vi "Write appender queue.vi"(8 "error in (no error)":errorcluster caption="에러 입력(에러 없음)", 10 "appender queue":refnum<queue>, 11 "GUI Log Class 입력":refnum<class "GUI Log Class.lvclass">) -> (0 "error out":errorcluster caption="에러 출력", 3 "GUI Log Class 출력":refnum<class "GUI Log Class.lvclass">)   [LabVIEW 2020, in "GUI Log Class.lvclass"]
uses:
  GUI Log Class.lvclass
  GUI Log Class.lvclass/GUI Log Class.ctl
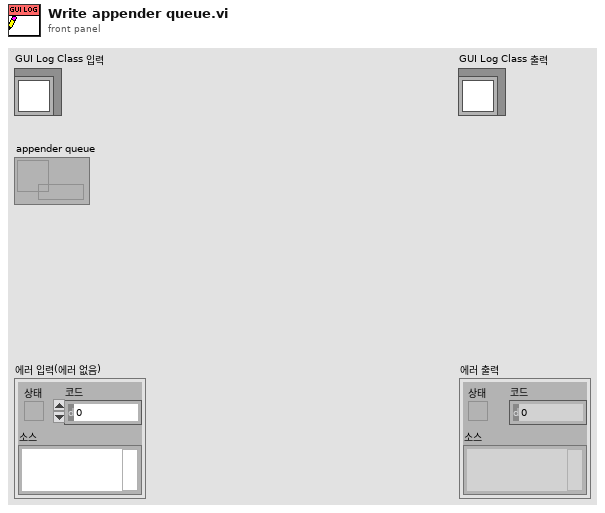
[diagram p1: front panel]
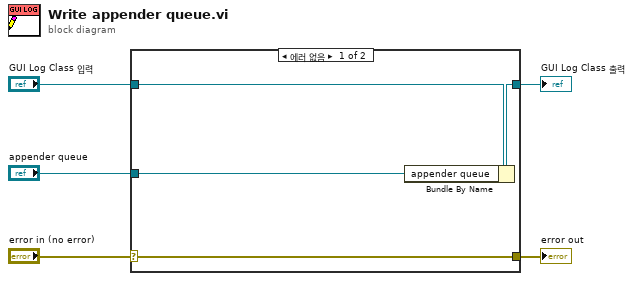
[diagram p0: block diagram]
diagram:
  n1 = case shown="에러 없음" "error in (no error)" {
    selector: "error in (no error)" -> [w9 w10]
    tunnel: [w9 w10] -> w4
    tunnel: [w7 w11] -> w2
    tunnel: "GUI Log Class 입력" -> [w8 w11]
    tunnel: "appender queue" -> [w6 _]
    frame No Error {
      n2 = Bundle By Name(cluster=w8, "appender queue"=w6) -> (w7:refnum<class "GUI Log Class.lvclass">)
    }
    frame Error {
    }
  }
  "error out" <- w4
  "GUI Log Class 출력" <- w2
